vi "SRV_Open TCP Connection.vi"(8 "error in (no error)":errorcluster, 11 "IP address":string) -> (0 "error out":errorcluster, 3 "connection ID":refnum<k5>)   [LabVIEW 2009]
doc: "Initialize a TCP Connection.\n\n\nModified for Benilde St. Margaret's School - Tim Jump\nBy Doug Schmertman - Logic PD\nCopyright 2012"
uses:
  SubVIs/SRVGlobals.vi
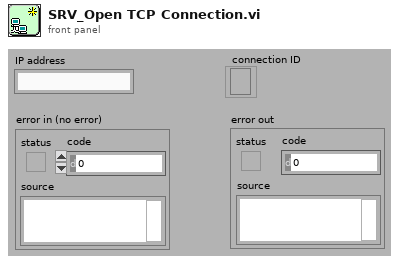
[diagram p1: front panel]
types:
  T1 = enum16{"Standard", "Buffered", "CRLF", "Immediate"}
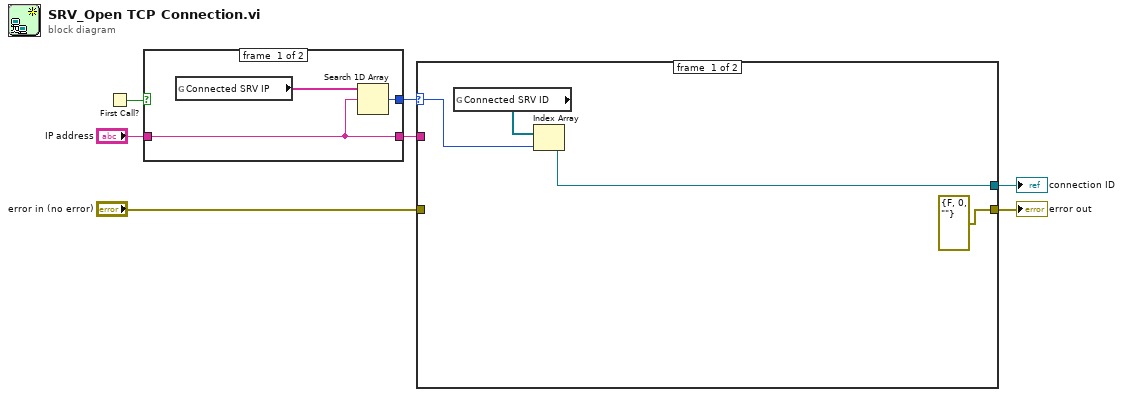
[diagram p0: block diagram]
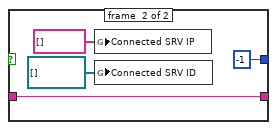
[diagram p2: hidden frame]
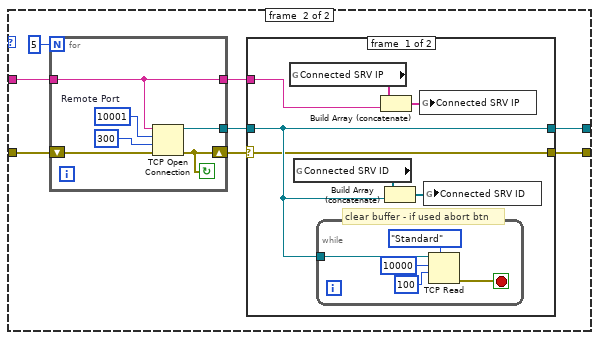
[diagram p3: hidden frame]
diagram:
  n1 = First Call?() -> (First Call?: T/F=w3:bool)
  n2 = case shown="False" w3 {
    tunnel: [w8 w11] -> w5
    tunnel: [w9 -1 ("index of element")] -> w4
    tunnel: "IP address" -> [w8 w11]
    frame #0 {
      n3 = global read "SRVGlobals.vi" "Connected SRV IP"() -> (w10:string[])
      n4 = Search 1D Array(1D array=w10, element=w8) -> (index of element=w9:i32)  [unwired: 1 in]
    }
    frame #1 {
      n5 = global write "SRVGlobals.vi" "Connected SRV IP"(string[] [] ("Connected SRV IP")) -> ()
      n6 = global write "SRVGlobals.vi" "Connected SRV ID"(refnum<k5>[] [] ("Connected SRV ID")) -> ()
    }
  }
  n7 = case shown="-1" w4 {
    selector: w4 -> [w18 _]
    tunnel: [w16 w21] -> w7
    tunnel: [errorcluster {"status"=FALSE, "code"=0, "source"=""} ("error out") w20] -> w6
    tunnel: w5 -> [_ w24]
    tunnel: "error in (no error)" -> [_ w19]
    frame #0 {
      n8 = global read "SRVGlobals.vi" "Connected SRV ID"() -> (w17:refnum<k5>[])
      n9 = Index Array(array=w17, index=w18) -> (element=w16:refnum<k5>)
    }
    frame #1 {
      n10 = for {
        N: 5 -> [_]
        tunnel: [w45] -> w23
        tunnel: w24 -> [w42]
        tunnel: [w42] -> w22
        shift-right: [w43] -> w25
        shift-left: w19 -> [w41]
        stop <- w43 continue-if-true
        w44 = u16 10001  # Remote Port
        n11 = TCP Open Connection ("TCP\n    Open Connection")(address=w42, remote port or service name=w44, timeout ms (60000)=300, error in (no error)=w41) -> (connection ID=w45:refnum<k5>, error out=w43:errorcluster)  [unwired: 1 in]
      }
      n12 = case shown="No Error" w25 {
        selector: w25 -> [w27 w39]
        tunnel: w22 -> [w32 _]
        tunnel: w23 -> [w28 w40]
        tunnel: [w28 w40] -> w21
        tunnel: [w27 w39] -> w20
        frame #0 {
          # "clear buffer - if used abort btn"
          n13 = global read "SRVGlobals.vi" "Connected SRV IP"() -> (w33:string[])
          n14 = global read "SRVGlobals.vi" "Connected SRV ID"() -> (w29:refnum<k5>[])
          n15 = while {
            tunnel: w28 -> [w34]
            stop <- w38 stop-if-true
            n16 = TCP Read(connection ID=w34, bytes to read=10000, 7:T1."Standard" ("mode (standard)"), 9:100 ("timeout ms (25000)")) -> (error out=w38:errorcluster)  [unwired: 1 in, 2 out]
          }
          n17 = Build Array (concatenate)(w33, w32) -> (w31:string[])
          n18 = Build Array (concatenate)(w29, w28) -> (w30:refnum<k5>[])
          n19 = global write "SRVGlobals.vi" "Connected SRV IP"(w31) -> ()
          n20 = global write "SRVGlobals.vi" "Connected SRV ID"(w30) -> ()
        }
        frame #1 {
        }
      }
    }
  }
  "error out" <- w6
  "connection ID" <- w7
